vi "Do Action.vi"(8 "error in (no error)":errorcluster, 9 "Display Queue":refnum<queue>, 10 "tlc_User Event Reference.ctl":T1, 11 "Application Command in":refnum<class "Application Command.lvclass">) -> (0 "error out":errorcluster)   [LabVIEW 2010, in "Application Command.lvclass"]
doc: "Do Action.vi for Application Command.lvclass has no functionality beyond defining the I/O for the child classes of Application Command.lvclass. Each child class will overwrite the functionality of this inherited method. These methods will be used to perform whatever functionality was previously within the consumer loop of TLC Main.vi.\n\nWhen called, the specific class type of Application Command in (Play, Load, Record, etc) will determine which specific version of Do Action.vi will be called."
uses:
  Application Command.lvclass
  Controls/tlc_User Interface Command.ctl
  Controls/tlc_User Interface Data Type.ctl
  Controls/tlc_User Event Reference.ctl
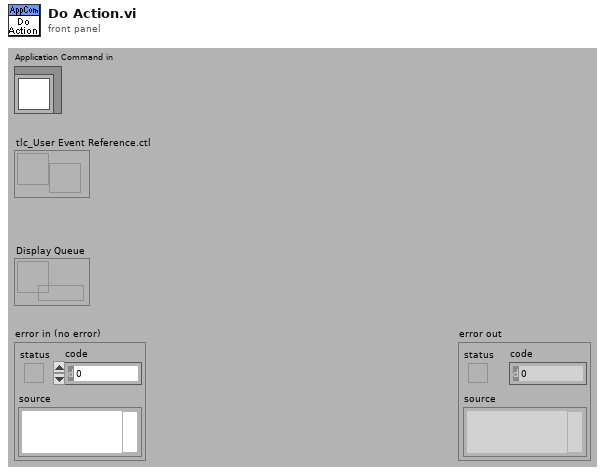
[diagram p1: front panel]
types:
  T1 = typedef "tlc_User Event Reference.ctl" = refnum<user-event>
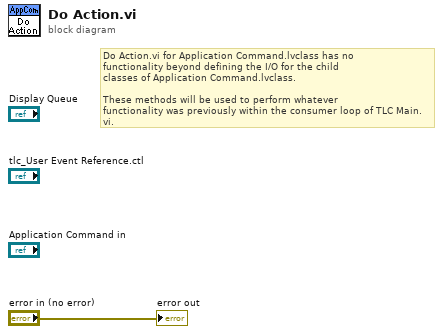
[diagram p0: block diagram]
diagram:
  # "Do Action.vi for Application Command.lvclass has no \nfunctionality beyond defining the I/O for the child \nclasses of Application Command.lvclass.  \n\nThese methods will be used to perform whatever \nfunctionality was previously within the consumer loop of TLC Main.vi."
  "error out" <- "error in (no error)"
